vi "Client Single Connection.vi"(8 "error in":errorcluster) -> ()   [LabVIEW 2020]
doc: "This WebSockets API example VI acts as a client to make an outgoing websockets connection. Receives/sends string data to the connected server.\nWebSockets 2.0.1.40\nSam Sharp - MediaMongrels Ltd\nCopyright (c) 2019, MediaMongrels Ltd"
uses:
  <vilib>/mediamongrels ltd/websockets/websockets/websocket/WebSocket.lvclass/WebSocket.ctl
  d81540a9-831c-486e-b785-0c0feae20dfe.vi
  <vilib>/mediamongrels ltd/websockets/websockets/WebSocket Client/WebSocket Client.lvclass
  C:/Program Files (x86)/National Instruments/LabVIEW 2020/vi.lib/mediamongrels ltd/websockets/websockets/websocket/WebSocket.lvclass
  <vilib>/Rock Robotics/Network Tables/NT Write Number.vi
  Framework/Robot Global Data.vi
  <vilib>/mediamongrels ltd/websockets/websockets/websocket/WebSocket.lvclass
panel:
  out "HTTP Headers 3":variant
  out "/limelight/":dbl[](array[numeric])
  out "Received Data":string
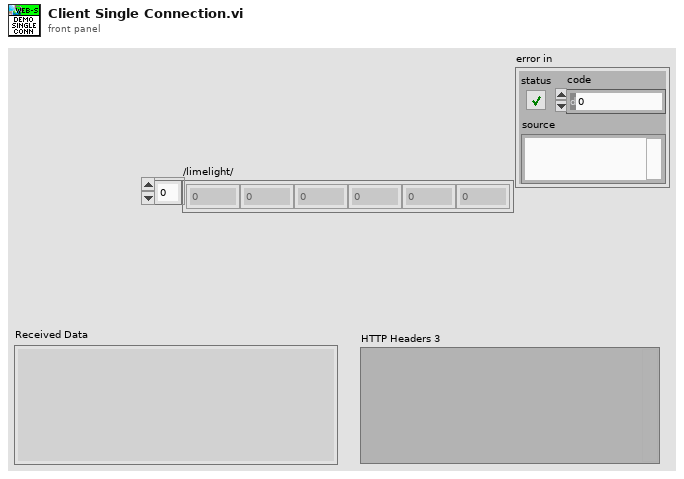
[diagram p1: front panel]
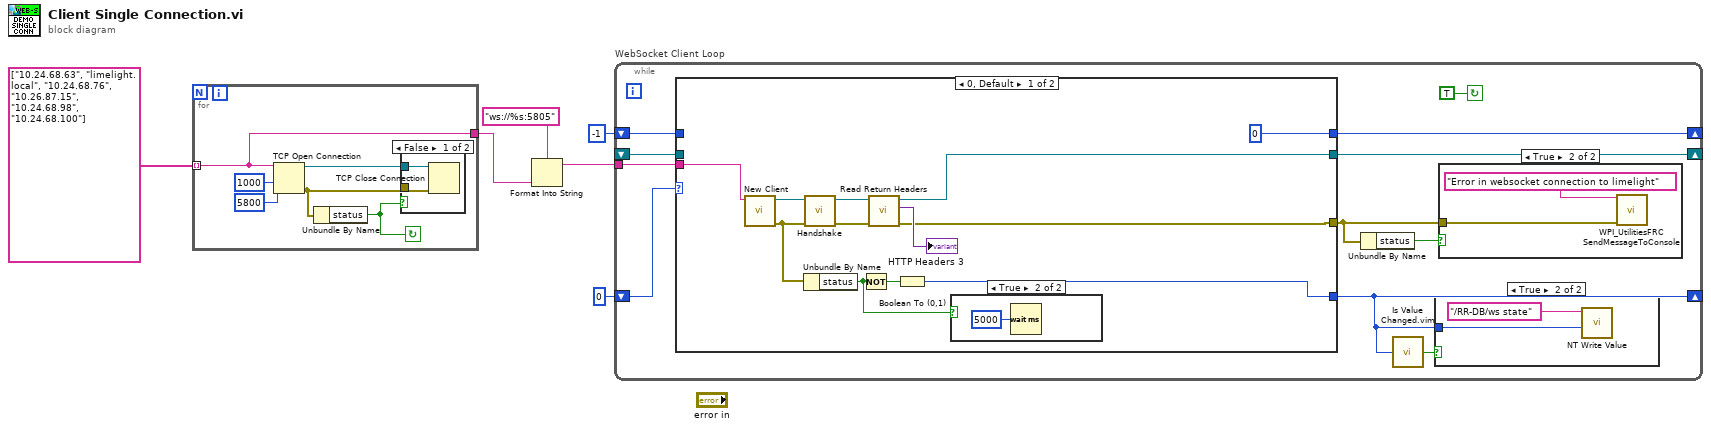
[diagram p0: block diagram]
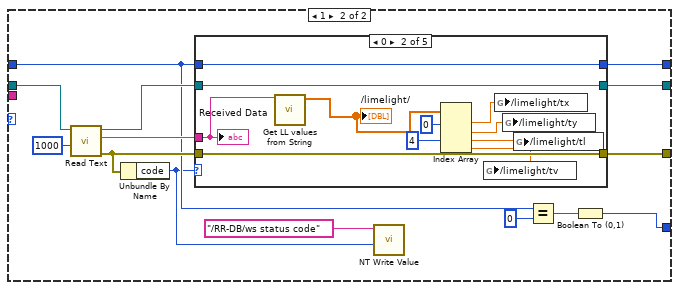
[diagram p6: hidden frame]
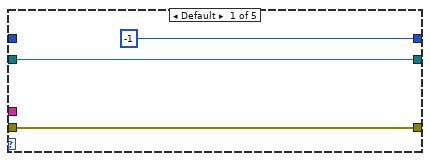
[diagram p7: hidden frame]
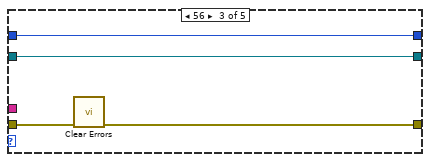
[diagram p8: hidden frame]
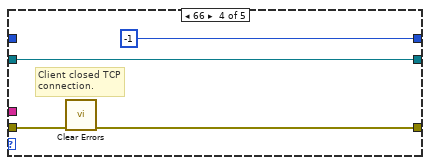
[diagram p9: hidden frame]
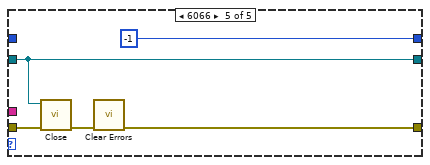
[diagram p10: hidden frame]
diagram:
  n1 = for {
    tunnel: string[] ["10.24.68.63", "limelight.local", "10.24.68.76", "10.26.87.15", "10.24.68.98", "10.24.68.100"] ("appended array") -> [w10] mode=indexing
    tunnel: [w10] -> w3
    stop <- w7 continue-if-true
    n2 = TCP Open Connection(address=w10, remote port or service name=u16 5800, timeout ms (60000)=1000) -> (connection ID=w11:refnum<k5>, error out=w9:errorcluster)  [unwired: 2 in]
    n3 = Unbundle By Name(w9) -> ("status"=w7:bool)
    n4 = case shown="False" w7 {
      tunnel: w11 -> [w14 _]
      tunnel: w9 -> [w13 _]
      frame False {
        n5 = TCP Close Connection(connection ID=w14, error in (no error)=w13) -> ()  [unwired: 1 in, 2 out]
      }
      frame True {
      }
    }
  }
  n6 = Format Into String(format string="ws://%s:5805" ("initial string"), w3) -> (resulting string=w2:string)  [unwired: 2 in, 1 out]
  n7 = while "WebSocket Client Loop" {
    shift-right: [w25] -> _
    shift-left: _ -> [w24]
    shift-right: [w23] -> _
    shift-left: -1 -> [w22]
    shift-right: [w16] -> _
    shift-left: 0 -> [w21]
    tunnel: w2 -> [w20]
    stop <- TRUE continue-if-true
    n8 = case shown="0, Default" w21 {
      tunnel: [w35 w56] -> w18
      tunnel: [w36 w55] -> w25
      tunnel: w24 -> [_ w54]
      tunnel: [0 w53] -> w23
      tunnel: w22 -> [_ w48]
      tunnel: [w31 w45] -> w16
      tunnel: w20 -> [w34 _]
      frame 0, Default {
        n9 = call <vilib>:"New Client.vi"("WebSocket URL"=w34) -> ("error out"=w33:errorcluster, "WebSocket Client out"=w40:refnum<class "WebSocket Client.lvclass">)  [unwired: 9 in]
        n10 = Unbundle By Name(w33) -> ("status"=w30:bool)
        n11 = call-dynamic "Handshake.vi"("error in (no error)"=w33, "WebSocket Client in"=w40) -> ("error out"=w39:errorcluster, "WebSocket Client out"=w38:refnum<class "WebSocket Client.lvclass">)  [unwired: 8 in]
        n12 = Not(x=w30) -> (.not. x?=w32:bool)
        n13 = call <vilib>:"Read Return Headers.vi"("error in (no error)"=w39, "WebSocket in"=w38) -> ("error out"=w35:errorcluster, "Return Headers"=→"HTTP Headers 3":variant, "WebSocket out"=w36:refnum<class "WebSocket Client.lvclass">)  [unwired: 7 in]
        n14 = Boolean To (0,1)(Boolean=w32) -> (0, 1=w31:i16)
        n15 = case shown="True" w30 {
          frame False {
          }
          frame True {
            n16 = Wait (ms)(milliseconds to wait=u32 5000) -> ()  [unwired: 1 out]
          }
        }
      }
      frame 1 {
        n17 = call-dynamic "Read Text.vi"("timeout ms (5000)"=1000, "WebSocket in"=w54) -> ("error out"=w50:errorcluster, "Data"=w51:string, "WebSocket out"=w49:refnum<class "WebSocket Client.lvclass">)  [unwired: 7 in]
        n18 = Unbundle By Name(w50) -> ("code"=w44:i32)
        n19 = case shown="0" w44 {
          tunnel: w51 -> [_ w67 _ _ _]
          tunnel: [w59 w70 w73 w75 w79] -> w56
          tunnel: w50 -> [w59 w70 w74 w78 w83]
          tunnel: w49 -> [w58 w69 w72 w77 w81]
          tunnel: [w58 w69 w72 w77 w81] -> w55
          tunnel: w48 -> [_ w68 w71 _ _]
          tunnel: [-1 w68 w71 -1 -1] -> w53
          frame Default {
          }
          frame 0 {
            n20 = call "Get LL values from String.vi"("input string"=w67) -> ("/limelight/"=w66:dbl[])  [unwired: 10 in]
            "/limelight/" <- w66
            n21 = Index Array(array=w66, index #1=0 ("index"), index #3=4 ("index")) -> (element #1=w63:dbl, element #2=w62:dbl, element #3=w60:dbl, element #4=w61:dbl)  [unwired: 2 in]
            n22 = global write "Robot Global Data.vi" "/limelight/tv"(w61) -> ()
            n23 = global write "Robot Global Data.vi" "/limelight/tx"(w63) -> ()
            n24 = global write "Robot Global Data.vi" "/limelight/ty"(w62) -> ()
            n25 = global write "Robot Global Data.vi" "/limelight/tl"(w60) -> ()
            "Received Data" <- w67
          }
          frame 56 {
            n26 = call <vilib>:"Clear Errors.vi"("error in (no error)"=w74) -> ("error out"=w73:errorcluster)  [unwired: 5 in, 1 out]
          }
          frame 66 {
            # "Client closed TCP connection."
            n27 = call <vilib>:"Clear Errors.vi"("error in (no error)"=w78) -> ("error out"=w75:errorcluster)  [unwired: 5 in, 1 out]
          }
          frame 6066 {
            n28 = call-dynamic "Close.vi"("error in (no error)"=w83, "WebSocket in"=w81) -> ("error out"=w82:errorcluster)  [unwired: 9 in]
            n29 = call <vilib>:"Clear Errors.vi"("error in (no error)"=w82) -> ("error out"=w79:errorcluster)  [unwired: 5 in, 1 out]
          }
        }
        n30 = call-poly <vilib>:"NT Write Value.vi"("Numeric"=w44, "Name"="/RR-DB/ws status code") -> ()  [unwired: 9 in, 1 out]
        n31 = Equal?(x=w48, y=0) -> (x = y?=w46:bool)
        n32 = Boolean To (0,1)(Boolean=w46) -> (0, 1=w45:i16)
      }
    }
    n33 = Unbundle By Name(w18) -> ("status"=w17:bool)
    n34 = call "Is Value Changed.vim"("value"=w16) -> ("changed or first call?"=w15:bool)
    n35 = case shown="True" w15 {
      tunnel: w16 -> [_ w26]
      frame False {
      }
      frame True {
        n36 = call-poly <vilib>:"NT Write Value.vi"("Numeric"=w26, "Name"="/RR-DB/ws state") -> ()  [unwired: 9 in, 1 out]
      }
    }
    n37 = case shown="True" w17 {
      tunnel: w18 -> [_ w28]
      frame False {
      }
      frame True {
        n38 = call <vilib>:"WPI_UtilitiesFRC SendMessageToConsole.vi"("Message"="Error in websocket connection to limelight", "error in (no error)"=w28) -> ()  [unwired: 13 in, 1 out]
      }
    }
  }
